vi "Settings Dialog.vi"(8 "error in (no error)":cluster{"状态":bool, "代码":i32, "源":string} caption="错误输入（无错误）", 11 "配置输入":T1={"硬件配置"={"硬件引用句柄<替换此项>"="", "信号类型<替换该项>"=enum."Sine Wave"}, "分析配置"={"统计"=TRUE}, "新采集到数据时如何操作"=enum."Replace"}) -> (0 "error out":cluster{"状态":bool, "代码":i32, "源":string} caption="错误输出", 2 "需要刷新UI？":bool, 3 "配置输出":T1={"硬件配置"={"硬件引用句柄<替换此项>"="", "信号类型<替换该项>"=enum."Sine Wave"}, "分析配置"={"统计"=TRUE}, "新采集到数据时如何操作"=enum."Replace"})   [LabVIEW 2013]
doc: "用于选择用户设置的对话框。"
uses:
  controls/User Specified Data.ctl
  controls/HW Configuration.ctl
  controls/Simulated Signal Type.ctl
  controls/Analysis Configuration.ctl
  controls/New Data Behavior.ctl
panel:
  in  "信号类型":u16(ring) items=["正弦波", "方波"]
  in  "新采集到数据时如何操作":u16(ring) items=["替换", "叠加", "添加"]
  in  "取消按钮":bool
  in  "确定按钮":bool
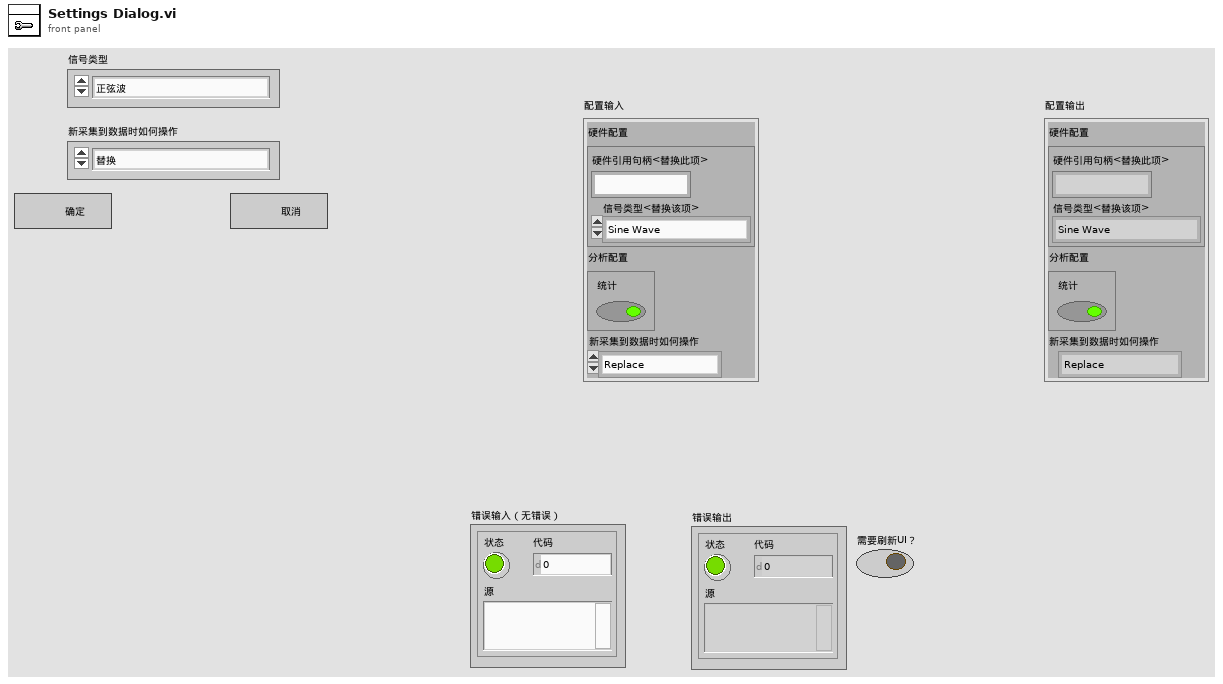
[diagram p1: front panel]
types:
  T1 = typedef "User Specified Data.ctl" = cluster{"硬件配置":T2, "分析配置":T4, "新采集到数据时如何操作":T5}
  T2 = typedef "HW Configuration.ctl" = cluster{"硬件引用句柄<替换此项>":string, "信号类型<替换该项>":T3}
  T3 = typedef "Simulated Signal Type.ctl" = enum16{"Sine Wave", "Square Wave"}
  T4 = typedef "Analysis Configuration.ctl" = cluster{"统计":bool}
  T5 = typedef "New Data Behavior.ctl" = enum16{"Replace", "Overlay", "Append"}
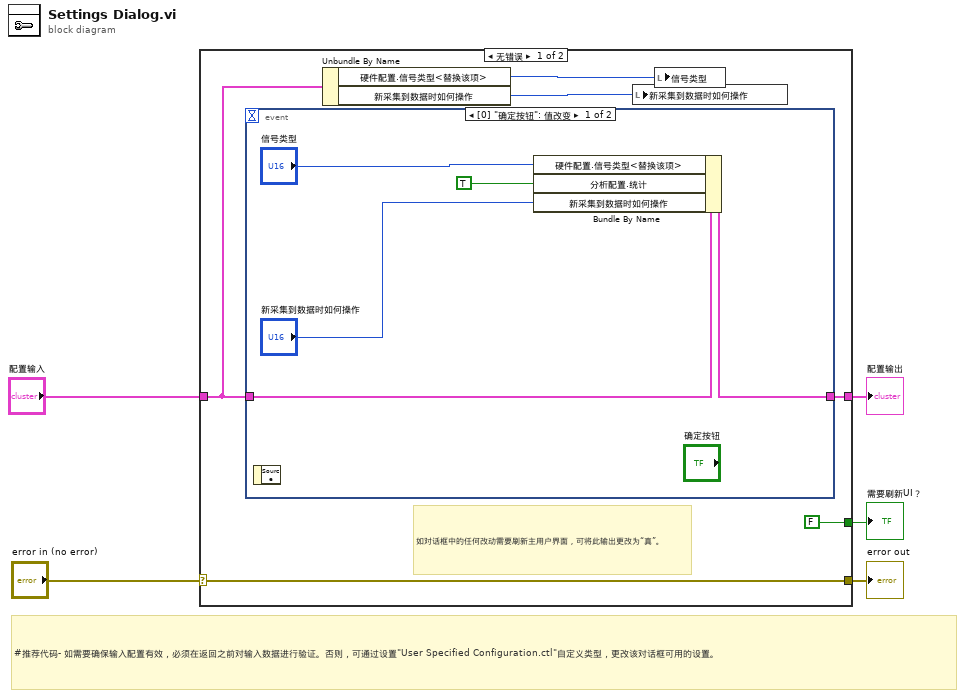
[diagram p0: block diagram]
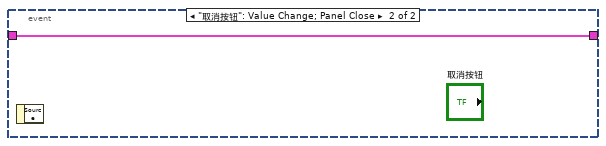
[diagram p2: hidden frame]
diagram:
  # "#推荐代码- 如需要确保输入配置有效，必须在返回之前对输入数据进行验证。否则，可通过设置\"User Specified Configuration.ctl\"自定义类型，更改该对话框可用的设置。"
  n1 = case shown="无错误" "error in (no error)" {
    selector: "error in (no error)" -> [w11 w19]
    tunnel: [w11 w19] -> w4
    tunnel: "配置输入" -> [w8 w18]
    tunnel: [w10 w18] -> w2
    tunnel: [FALSE ("UI Refresh Needed?") _] -> w1
    frame No Error {
      # "如对话框中的任何改动需要刷新主用户界面，可将此输出更改为“真”。"
      n2 = event shown="[0] \"确定按钮\": 值改变" {
        selector: _ -> [_ _]
        dyn-events: _ -> [_ _]
        timeout: _ -> [_ _]
        tunnel: [w15 w17] -> w10
        tunnel: w8 -> [w16 w17]
        event "确定按钮": Value Change {
          n3 = event-data() -> ()  [unwired: 1 in, 1 out]
          n4 = Bundle By Name(cluster=w16, "硬件配置.信号类型<替换该项>"="信号类型", "分析配置.统计"=TRUE ("Analysis Configuration.Statistics"), "新采集到数据时如何操作"="新采集到数据时如何操作") -> (w15:T1)
        }
        event "取消按钮": Value Change; Panel Close {
          n5 = event-data() -> ()  [unwired: 1 in, 1 out]
        }
      }
      n6 = Unbundle By Name(w8) -> ("硬件配置.信号类型<替换该项>"=w7:T3, "新采集到数据时如何操作"=w6:T5)
      n7 = local write "新采集到数据时如何操作"(w6) -> ()
      n8 = local write "信号类型"(w7) -> ()
    }
    frame Error {
    }
  }
  "需要刷新UI？" <- w1
  "error out" <- w4
  "配置输出" <- w2
